vi "Background voltage.vi"(8 "error in (no error)":errorcluster, 10 "Final number of points":dbl, 11 "data array":dbl[](array[numeric])) -> (0 "error out":errorcluster, 3 "Background level (V)":dbl)   [LabVIEW 2017, in "Processing.lvlib"]
doc: "Calculates the ambient voltage from 75% of the pretrigger data (pretrigger = 10% of \nthe full dataset), i.e. it's calculated from the first 7.5% of the data"
uses:
  Processing.lvlib
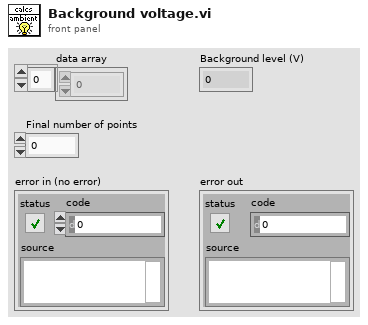
[diagram p1: front panel]
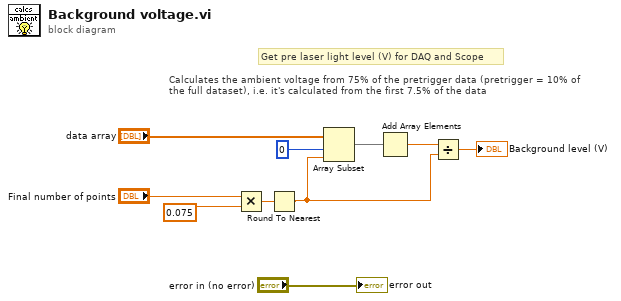
[diagram p0: block diagram]
diagram:
  # "Calculates the ambient voltage from 75% of the pretrigger data (pretrigger = 10% of \nthe full dataset), i.e. it's calculated from the first 7.5% of the data"
  # "Get pre laser light level (V) for DAQ and Scope"
  n1 = Multiply(x="Final number of points", y=0.075) -> (x*y=w4:dbl)
  n2 = Round To Nearest(number=w4) -> (nearest integer value=w3:dbl)
  n3 = Array Subset(array="data array", index=0, length=w3) -> (w7:dbl[])
  n4 = Add Array Elements(numeric array=w7) -> (sum=w6:dbl)
  n5 = Divide(x=w6, y=w3) -> (x/y=→"Background level (V)":dbl)
  "error out" <- "error in (no error)"
